vi "Shift Register Demo - Past values.vi"() -> ()   [LabVIEW 2011]
panel:
  out "N":i32
  out "n-3":i32
  out "n-1":i32
  out "n-1":i32
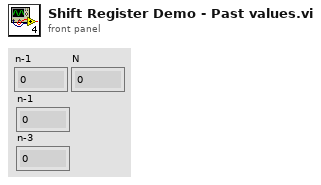
[diagram p1: front panel]
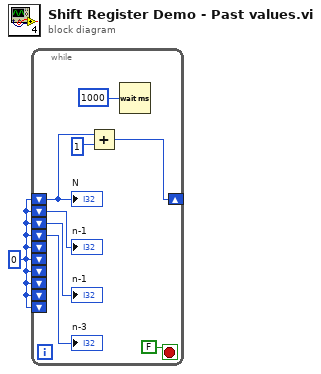
[diagram p0: block diagram]
diagram:
  w1 = 0
  n1 = while {
    shift-right: [w3] -> _
    shift-left: w1 -> [w8]
    shift-left: w1 -> [w6]
    shift-left: w1 -> [w5]
    shift-left: w1 -> [w4]
    shift-left: w1 -> [_]
    shift-left: w1 -> [_]
    shift-left: w1 -> [_]
    shift-left: w1 -> [_]
    shift-left: w1 -> [_]
    shift-left: w1 -> [_]
    stop <- FALSE stop-if-true
    n2 = Add(x=w8, y=1) -> (x+y=w3:i32)
    n3 = Wait (ms)(milliseconds to wait=u32 1000) -> ()  [unwired: 1 out]
    "n-1" <- w6
    "n-1" <- w5
    "n-3" <- w4
    "N" <- w8
  }
